vi "ExtractMeasurementDataFromCOMbuffer.vi"(8 "error in (no error)":errorcluster, 11 "Input OPC data":string) -> (0 "error out":errorcluster, 2 "Valid Data":bool, 3 "Output Number of Particles per 100 CC":i32[](array[numeric]))   [LabVIEW 2013]
doc: "Use this template to build a VI to use as a subVI."
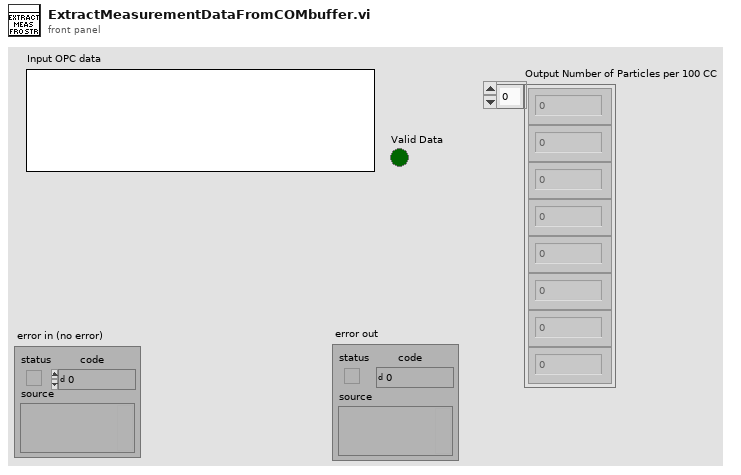
[diagram p1: front panel]
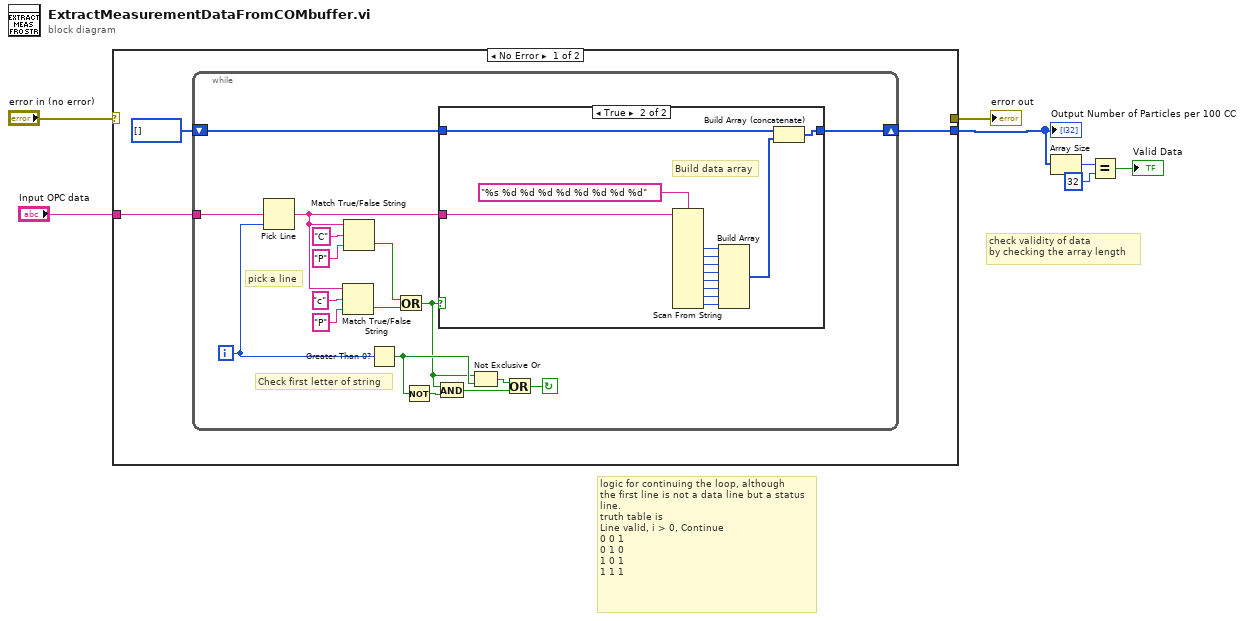
[diagram p0: block diagram]
diagram:
  # "logic for continuing the loop, although\nthe first line is not a data line but a status\nline.\ntruth table is \nLine valid, i > 0, Continue\n0 0 1\n0 1 0\n1 0 1\n1 1 1"
  # "check validity of data\nby checking the array length"
  n1 = case shown="No Error" "error in (no error)" {
    selector: "error in (no error)" -> [_ w42]
    tunnel: [_ w42] -> w6
    tunnel: "Input OPC data" -> [w10 _]
    tunnel: [w8 _] -> w4
    frame No Error {
      n2 = while {
        tunnel: w10 -> [w18]
        shift-right: [w19] -> w8
        shift-left: i32[] [] ("Output Number of Particles per 100 CC") -> [w20]
        i -> [w17]
        stop <- w11 continue-if-true
        # "pick a line"
        # "Check first letter of string"
        n3 = Pick Line(multi-line string=w18, line index=w17) -> (output string=w21:string)  [unwired: 1 in]
        n4 = Match True/False String(2:"P" ("false string"), 3:"c" ("true string"), 4:w21) -> (0:w27:bool)  [unwired: 1 out]
        n5 = Match True/False String(2:"P" ("false string"), 3:"C" ("true string"), 4:w21) -> (0:w24:bool)  [unwired: 1 out]
        n6 = Greater Than 0?(x=w17) -> (x > 0?=w15:bool)
        n7 = Or(x=w24, y=w27) -> (x .or. y?=w14:bool)
        n8 = Not(x=w15) -> (.not. x?=w16:bool)
        n9 = And(x=w14, y=w16) -> (x .and. y?=w12:bool)
        n10 = case shown="True" w14 {
          tunnel: w21 -> [_ w33]
          tunnel: w20 -> [w28 w31]
          tunnel: [w28 w29] -> w19
          frame False {
          }
          frame True {
            # "Build data array"
            n11 = Scan From String(format string="%s %d %d %d %d %d %d %d %d", input string=w33) -> (output 2=w34:i32, output 3=w35:i32, output 4=w36:i32, output 5=w37:i32, output 6=w38:i32, output 7=w39:i32, output 8=w40:i32, output 9=w41:i32)  [unwired: 12 in, 3 out]
            n12 = Build Array(w34, w35, w36, w37, w38, w39, w40, w41) -> (w30:i32[])
            n13 = Build Array (concatenate)(w31, w30) -> (w29:i32[])
          }
        }
        n14 = Not Exclusive Or(1:w15, 2:w14) -> (0:w13:bool)
        n15 = Or(x=w13, y=w12) -> (x .or. y?=w11:bool)
      }
    }
    frame Error {
    }
  }
  "error out" <- w6
  "Output Number of Particles per 100 CC" <- w4
  n16 = Array Size(array=w4) -> (size(s)=w3:i32)
  n17 = Equal?(x=w3, y=32) -> (x = y?=→"Valid Data":bool)
